vi "Blynk Notify.vi"(6 "message":string, 8 "error in (no error)":errorcluster, 11 "connection":refnum<k5>) -> (0 "error out":errorcluster, 3 "connection out":refnum<k5>)   [LabVIEW 2014]
uses:
  utilities/MsgType.ctl
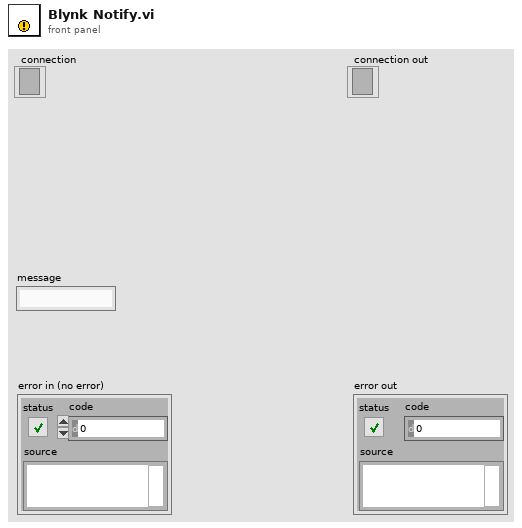
[diagram p1: front panel]
types:
  T1 = typedef "MsgType.ctl" = enum8{"RSP", "REGISTER", "LOGIN", "SAVE_PROF", "LOAD_PROF", "GET_TOKEN", "PING", "ACTIVATE", "DEACTIVATE", "REFRESH", "UNDEFINED0", "UNDEFINED1", "TWEET", "EMAIL", "NOTIFY", "BRIDGE", "UNDEFINED2", "UNDEFINED3", "UNDEFINED4", "UNDEFINED5", "HW"}
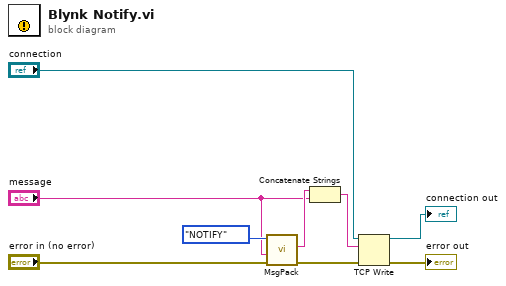
[diagram p0: block diagram]
diagram:
  n1 = call "MsgPack.vi"("error in"="error in (no error)", "msg"="message", "msg_type"=MsgType."NOTIFY") -> ("error out"=w2:errorcluster, "msg_data"=w8:string)  [unwired: 7 in]
  n2 = Concatenate Strings(w8, "message") -> (w9:string)
  n3 = TCP Write(connection ID="connection", data in=w9, error in (no error)=w2) -> (connection ID out=→"connection out":refnum<k5>, error out=→"error out":errorcluster)  [unwired: 1 in, 1 out]
